vi "Get Window Title.vi"(8 "error in (no error)":errorcluster, 11 "hwnd":u32) -> (0 "error out":errorcluster, 3 "Window Title":string)   [LabVIEW 2019, in "LV MDI.lvclass"]
doc: "Copies the text of the specified window's title bar (if it has one) into a buffer."
uses:
  LV MDI.lvclass
  user32.dll
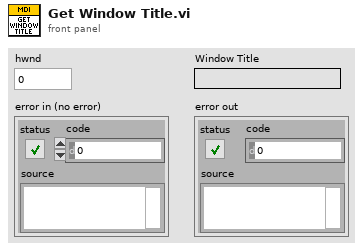
[diagram p1: front panel]
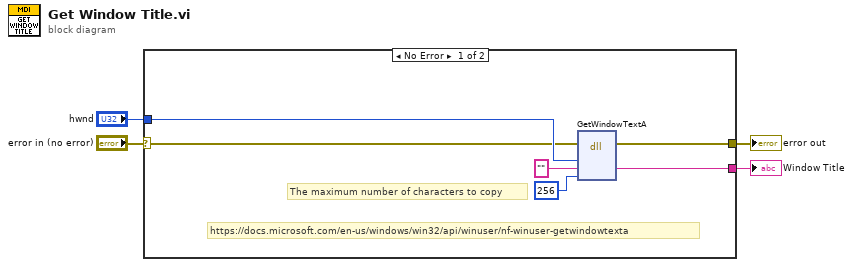
[diagram p0: block diagram]
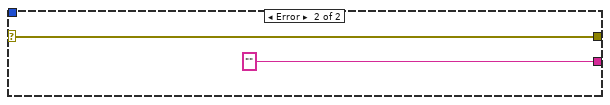
[diagram p2: hidden frame]
diagram:
  n1 = case shown="No Error" "error in (no error)" {
    selector: "error in (no error)" -> [w7 w12]
    tunnel: "hwnd" -> [w8 _]
    tunnel: [w6 w12] -> w2
    tunnel: [w5 "" ("lpString")] -> w1
    frame No Error {
      # "https://docs.microsoft.com/en-us/windows/win32/api/winuser/nf-winuser-getwindowtexta"
      # "The maximum number of characters to copy"
      n2 = dll-call lib="user32.dll" fn="GetWindowTextA"(error in=w7, "hwnd"=w8, "lpString"="", "nMaxcount"=256) -> (error out=w6:errorcluster, "lpString"=w5:string)  [unwired: 5 in, 1 out]
    }
    frame Error {
    }
  }
  "error out" <- w2
  "Window Title" <- w1
